vi "Untitled 1.vi"() -> ()   [LabVIEW 2021]
uses:
  1a71aa08-014e-3fd2-ac8a-803d5703e53f.vi
  Table/Table.lvclass
panel:
  in  "Numeric":dbl
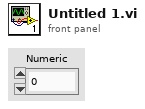
[diagram p1: front panel]
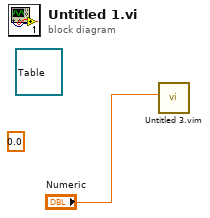
[diagram p0: block diagram]
diagram:
  (unwired) 0.0 ("Numeric")
  (unwired) refnum<class "Table.lvclass"> refnum ("Table in")
  n1 = call "Untitled 3.vim"("Numeric"="Numeric") -> ()  [unwired: 7 in, 3 out]
